vi "net_cycle_thread.vi"() -> ()   [LabVIEW 2020]
doc: "该模板用于创建生产者／消费者模式的应用程序，以事件驱动的方式，生成队列中的项。如需通过响应事件实现代码的异步执行，同时不影响用户界面的响应速度，可考虑用该模式替代“用户界面事件处理器”模式。"
uses:
  <vilib>/Instr/_visa.llb/VISA Configure Serial Port (Instr).vi
panel:
  out "转发标志1":bool
  out "发送字节数1":u32
  out "转发标志3":bool
  out "发送字节数3":u32
  out "转发标志2":bool
  out "发送字节数2":u32
  out "开启计时器 3":u32
  out "开启计时器 2":u32
  out "开启计时器":u32
  in  "关时长(ms) 3":u32
  out "数据接收 3":string
  in  "读取的字节 3":i32=500
  in  "远程端口或服务名称 3":u16=29000
  in  "远程主机地址3":string="192.168.76.100"
  in  "关时长(ms) 2":u32
  out "数据接收 2":string
  in  "读取的字节 2":i32=500
  in  "远程端口或服务名称 2":u16=28000
  in  "远程主机地址 2":string="192.168.76.200"
  in  "关时长(ms)":u32
  out "数据接收":string
  in  "读取标准码词":bool
  out "读取标准码词":string
  in  "发送数据(十六进制)":string="\u0001T\u0004"
  in  "读取的字节":i32=500
  in  "远程端口或服务名称":u16=30000
  in  "远程主机地址":string="192.168.76.172"
  in  "压缩机":bool
  in  "臭氧":bool
  in  "开时长(ms)":u32
  in  "开时长(ms) 2":u32
  in  "开时长(ms)  3":u32
  in  "开始测试":bool
  in  "风机":bool
  in  "继电器调试":bool
  in  "打开开关":bool
  in  "串口资源":refnum<visa-resource-name>
  in  "stop":bool caption="停止"
  out "错误输出":errorcluster
  out "error out":errorcluster caption="继电器板错误输入输出"
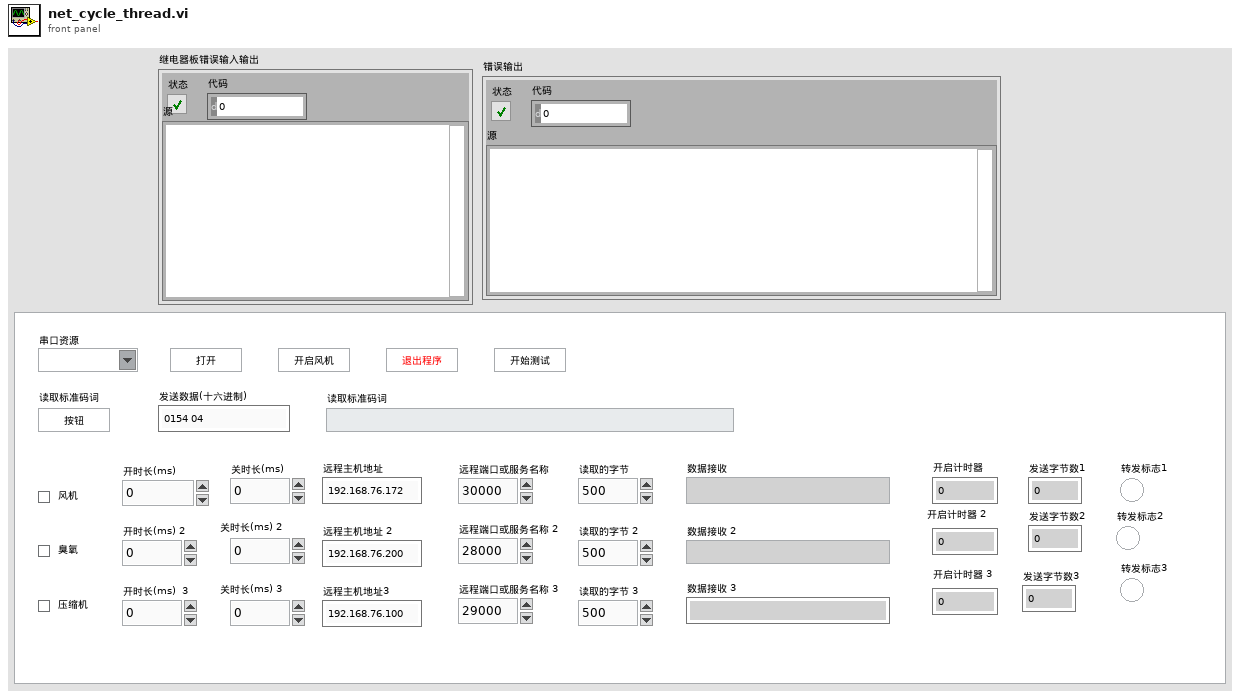
[diagram p1: front panel]
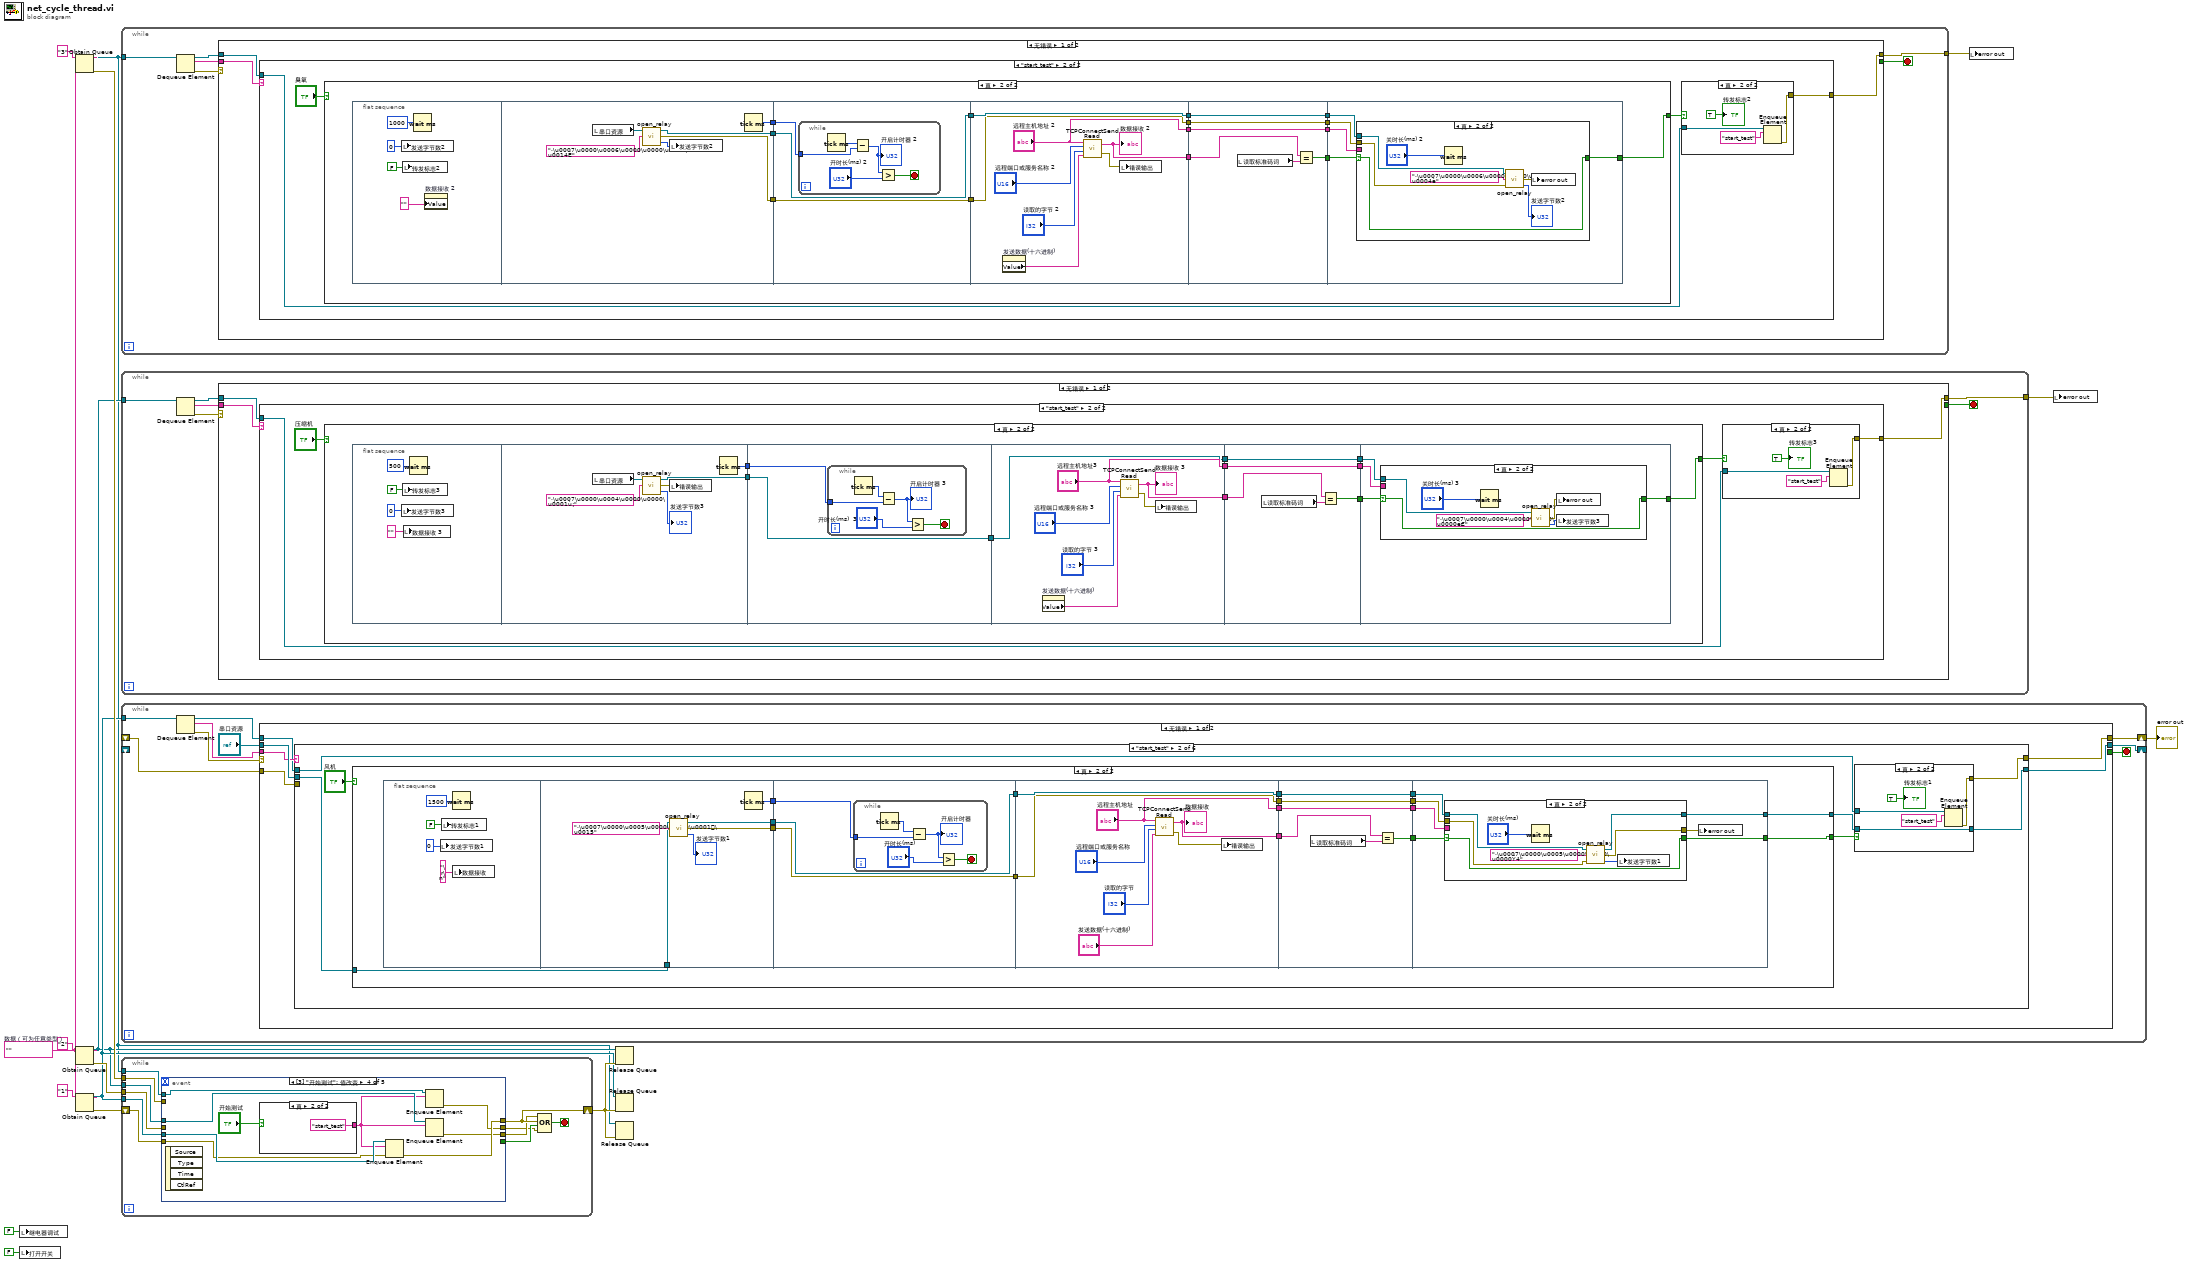
[diagram p0: block diagram]
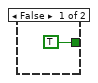
[diagram p4: hidden frame]
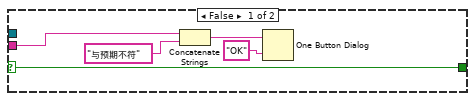
[diagram p5: hidden frame]
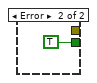
[diagram p6: hidden frame]
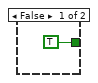
[diagram p9: hidden frame]
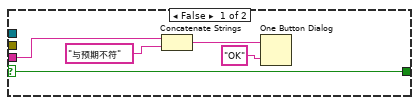
[diagram p10: hidden frame]
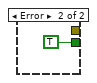
[diagram p11: hidden frame]
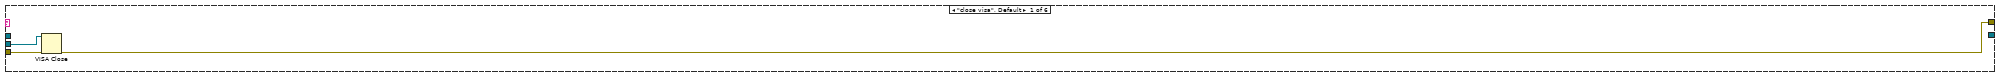
[diagram p12: hidden frame]
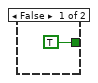
[diagram p14: hidden frame]
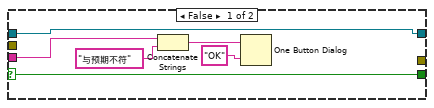
[diagram p15: hidden frame]
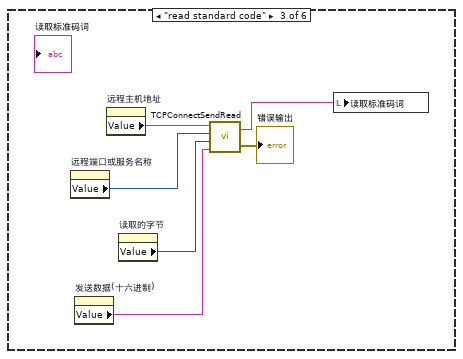
[diagram p16: hidden frame]
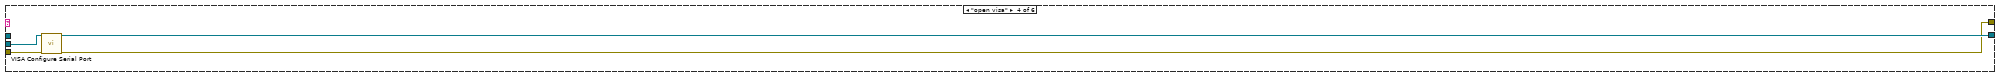
[diagram p17: hidden frame]
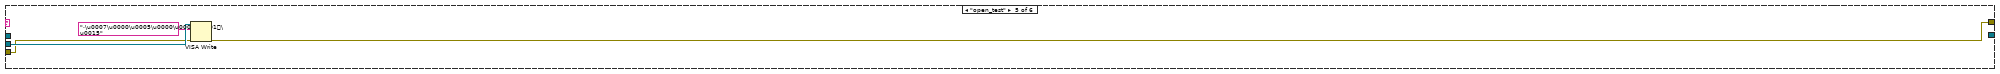
[diagram p18: hidden frame]
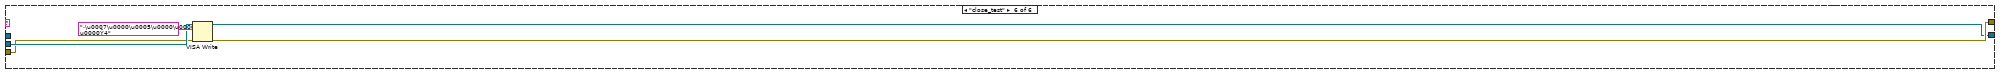
[diagram p19: hidden frame]
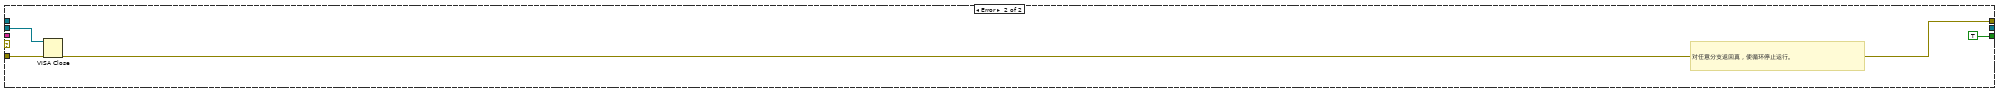
[diagram p20: hidden frame]
diagram:
  w12 = ""  # 数据（可为任意类型）
  n1 = local write "继电器调试"(FALSE ("继电器调试")) -> ()
  n2 = local write "打开开关"(FALSE ("打开开关")) -> ()
  n3 = Obtain Queue(name (unnamed)="3" ("名称（未命名）"), element data type=w12) -> (queue out=w3:refnum<queue>, error out=w11:errorcluster)  [unwired: 3 in, 1 out]
  n4 = Obtain Queue(name (unnamed)="2" ("名称（未命名）"), element data type=w12) -> (queue out=w4:refnum<queue>, error out=w10:errorcluster)  [unwired: 3 in, 1 out]
  n5 = Obtain Queue(name (unnamed)="1" ("名称（未命名）"), element data type=w12) -> (queue out=w8:refnum<queue>, error out=w16:errorcluster)  [unwired: 3 in, 1 out]
  n6 = while {
    tunnel: w3 -> [w19]
    tunnel: [w18] -> w1
    stop <- w20 stop-if-true
    n7 = Dequeue Element(queue=w19) -> (queue out=w17:refnum<queue>, element=w21:string, error out=w22:errorcluster)  [unwired: 2 in, 1 out]
    n8 = case shown="无错误" w22 {
      tunnel: w21 -> [w25 _]
      tunnel: [_ TRUE] -> w20
      tunnel: [w24 _] -> w18
      tunnel: w17 -> [w23 _]
      frame No Error {
        n9 = case shown="\"start_test\"" w25 {
          tunnel: [_ w27] -> w24
          tunnel: w23 -> [_ w26]
          frame "假", Default {
          }
          frame "start_test" {
            n10 = case shown="真" "臭氧" {
              tunnel: [TRUE w36] -> w28
              frame False {
              }
              frame True {
                n11 = flat-sequence {
                  tunnel: [w57] -> w48
                  tunnel: [w56] -> w40
                  tunnel: [w55] -> w35
                  tunnel: w48 -> [w61]
                  tunnel: [w61] -> w47
                  tunnel: [w60] -> w41
                  tunnel: w40 -> [w60]
                  tunnel: w35 -> [w59]
                  tunnel: w47 -> [w74]
                  tunnel: [w74] -> w46
                  tunnel: [w71] -> w45
                  tunnel: [w70] -> w42
                  tunnel: w41 -> [w70]
                  tunnel: ["远程主机地址 2"] -> w38
                  tunnel: w46 -> [w78]
                  tunnel: w45 -> [w80]
                  tunnel: [w78] -> w44
                  tunnel: [w77] -> w43
                  tunnel: w42 -> [w77]
                  tunnel: [w76] -> w39
                  tunnel: w38 -> [w76]
                  tunnel: [w75] -> w37
                  tunnel: w44 -> [w85]
                  tunnel: w43 -> [w84]
                  tunnel: w39 -> [w83]
                  tunnel: w37 -> [w82]
                  tunnel: [w81] -> w36
                  frame #0 {
                    n12 = local write "发送字节数2"(u32 0 ("发送字节数2")) -> ()
                    n13 = local write "转发标志2"(FALSE ("转发标志2")) -> ()
                    n14 = Wait (ms)(milliseconds to wait=u32 1000 ("等待时间（毫秒）")) -> ()  [unwired: 1 out]
                    n15 = property on="数据接收 2" class="Str"("Value"="" ("数据接收 2")) -> ()  [unwired: 2 in, 2 out]
                  }
                  frame #1 {
                    n16 = local read "串口资源"() -> (w54:refnum<visa-resource-name>)
                    n17 = call "open_relay.vi"("写入缓冲区"="·\u0007\u0000\u0006\u0000\u0000\u0001\u0014É", "VISA资源名称"=w54) -> ("返回数"=w53:u32, "错误输出"=w56:errorcluster, "VISA资源名称输出"=w57:refnum<visa-resource-name>)  [unwired: 1 in]
                    n18 = local write "发送字节数2"(w53) -> ()
                    n19 = Tick Count (ms)() -> (millisecond timer value=w55:u32)
                  }
                  frame #2 {
                    n20 = while {
                      tunnel: w59 -> [w64]
                      stop <- w65 stop-if-true
                      n21 = Tick Count (ms)() -> (millisecond timer value=w66:u32)
                      n22 = Subtract(x=w66, y=w64) -> (x-y=w63:u32)
                      "开启计时器 2" <- w63
                      n23 = Greater?(x=w63, y="开时长(ms) 2") -> (0:w65:bool)
                    }
                  }
                  frame #3 {
                    n24 = property on="发送数据(十六进制)" class="Str"() -> ("Value"=w69:string)  [unwired: 2 in, 2 out]
                    n25 = call "TCPConnectSendRead.vi"("数据输入"=w69, "读取的字节"="读取的字节 2", "远程端口或服务名称"="远程端口或服务名称 2", "地址"="远程主机地址 2") -> ("错误输出"=w67:errorcluster, "数据输出"=w71:string)
                    "数据接收 2" <- w71
                    n26 = local write "错误输出"(w67) -> ()
                  }
                  frame #4 {
                    n27 = local read "读取标准码词"() -> (w79:string)
                    n28 = Equal?(x=w80, y=w79) -> (x = y?=w75:bool)
                  }
                  frame #5 {
                    n29 = case shown="真" w82 {
                      selector: w82 -> [w86 w92]
                      tunnel: w85 -> [_ w96]
                      tunnel: w84 -> [_ w95]
                      tunnel: w83 -> [w87 _]
                      tunnel: [w86 w92] -> w81
                      frame False {
                        n30 = Concatenate Strings(w87, "与预期不符" ("字符串")) -> (w90:string)
                        n31 = One Button Dialog(message=w90, button name ("OK")="OK" ("按钮名称（“确定”）")) -> ()  [unwired: 1 out]
                      }
                      frame True {
                        n32 = Wait (ms)(milliseconds to wait="关时长(ms) 2") -> ()  [unwired: 1 out]
                        n33 = call "open_relay.vi"("错误输入（无错误）"=w95, "写入缓冲区"="·\u0007\u0000\u0006\u0000\u0000\u0000\u0004è", "VISA资源名称"=w96) -> ("返回数"=→"发送字节数2":u32, "错误输出"=w94:errorcluster)  [unwired: 1 out]
                        n34 = local write "error out"(w94) -> ()
                      }
                    }
                  }
                }
              }
            }
            n35 = case shown="真" w28 {
              tunnel: [_ w32] -> w27
              tunnel: w26 -> [_ w31]
              frame False {
              }
              frame True {
                n36 = Enqueue Element(queue=w31, element="start_test" ("元素")) -> (error out=w32:errorcluster)  [unwired: 2 in, 2 out]
                "转发标志2" <- TRUE ("转发标志2")
              }
            }
          }
        }
      }
      frame Error {
      }
    }
  }
  n37 = while {
    tunnel: w4 -> [w101]
    tunnel: [w100] -> w2
    stop <- w102 stop-if-true
    n38 = Dequeue Element(queue=w101) -> (queue out=w99:refnum<queue>, element=w103:string, error out=w104:errorcluster)  [unwired: 2 in, 1 out]
    n39 = case shown="无错误" w104 {
      tunnel: w103 -> [w107 _]
      tunnel: [_ TRUE] -> w102
      tunnel: [w106 _] -> w100
      tunnel: w99 -> [w105 _]
      frame No Error {
        n40 = case shown="\"start_test\"" w107 {
          tunnel: [_ w109] -> w106
          tunnel: w105 -> [_ w108]
          frame "假", Default {
          }
          frame "start_test" {
            n41 = case shown="真" "压缩机" {
              tunnel: [TRUE w122] -> w110
              frame False {
              }
              frame True {
                n42 = flat-sequence {
                  tunnel: [w135] -> w118
                  tunnel: [w134] -> w117
                  tunnel: [w138] -> w119
                  tunnel: w118 -> [w138]
                  tunnel: w117 -> [w137]
                  tunnel: [w146] -> w126
                  tunnel: ["远程主机地址3"] -> w123
                  tunnel: [w144] -> w120
                  tunnel: w119 -> [w144]
                  tunnel: w126 -> [w155]
                  tunnel: [w153] -> w125
                  tunnel: [w152] -> w124
                  tunnel: w123 -> [w152]
                  tunnel: [w151] -> w121
                  tunnel: w120 -> [w151]
                  tunnel: w125 -> [w159]
                  tunnel: w124 -> [w158]
                  tunnel: [w157] -> w122
                  tunnel: w121 -> [w156]
                  frame #0 {
                    n43 = local write "发送字节数3"(u32 0 ("返回数3")) -> ()
                    n44 = local write "转发标志3"(FALSE ("转发标志3")) -> ()
                    n45 = local write "数据接收 3"("" ("数据接收 3")) -> ()
                    n46 = Wait (ms)(milliseconds to wait=u32 500 ("等待时间（毫秒）")) -> ()  [unwired: 1 out]
                  }
                  frame #1 {
                    n47 = local read "串口资源"() -> (w133:refnum<visa-resource-name>)
                    n48 = call "open_relay.vi"("写入缓冲区"="·\u0007\u0000\u0004\u0000\u0000\u0001ù¡", "VISA资源名称"=w133) -> ("返回数"=→"发送字节数3":u32, "错误输出"=w132:errorcluster, "VISA资源名称输出"=w135:refnum<visa-resource-name>)  [unwired: 1 in]
                    n49 = local write "错误输出"(w132) -> ()
                    n50 = Tick Count (ms)() -> (millisecond timer value=w134:u32)
                  }
                  frame #2 {
                    n51 = while {
                      tunnel: w137 -> [w141]
                      stop <- w142 stop-if-true
                      n52 = Tick Count (ms)() -> (millisecond timer value=w143:u32)
                      n53 = Subtract(x=w143, y=w141) -> (x-y=w140:u32)
                      "开启计时器 3" <- w140
                      n54 = Greater?(x=w140, y="开时长(ms)  3") -> (0:w142:bool)
                    }
                  }
                  frame #3 {
                    n55 = property on="发送数据(十六进制)" class="Str"() -> ("Value"=w148:string)  [unwired: 2 in, 2 out]
                    n56 = call "TCPConnectSendRead.vi"("数据输入"=w148, "读取的字节"="读取的字节 3", "远程端口或服务名称"="远程端口或服务名称 3", "地址"="远程主机地址3") -> ("错误输出"=w147:errorcluster, "数据输出"=w146:string)
                    "数据接收 3" <- w146
                    n57 = local write "错误输出"(w147) -> ()
                  }
                  frame #4 {
                    n58 = local read "读取标准码词"() -> (w154:string)
                    n59 = Equal?(x=w155, y=w154) -> (x = y?=w153:bool)
                  }
                  frame #5 {
                    n60 = case shown="真" w159 {
                      selector: w159 -> [w160 w167]
                      tunnel: w158 -> [w161 _]
                      tunnel: [w160 w167] -> w157
                      tunnel: w156 -> [_ w166]
                      frame False {
                        n61 = Concatenate Strings(w161, "与预期不符" ("字符串")) -> (w162:string)
                        n62 = One Button Dialog(message=w162, button name ("OK")="OK" ("按钮名称（“确定”）")) -> ()  [unwired: 1 out]
                      }
                      frame True {
                        n63 = Wait (ms)(milliseconds to wait="关时长(ms) 3") -> ()  [unwired: 1 out]
                        n64 = call "open_relay.vi"("写入缓冲区"="·\u0007\u0000\u0004\u0000\u0000\u0000é€", "VISA资源名称"=w166) -> ("返回数"=w165:u32, "错误输出"=w169:errorcluster)  [unwired: 1 in, 1 out]
                        n65 = local write "error out"(w169) -> ()
                        n66 = local write "发送字节数3"(w165) -> ()
                      }
                    }
                  }
                }
              }
            }
            n67 = case shown="真" w110 {
              tunnel: [_ w114] -> w109
              tunnel: w108 -> [_ w113]
              frame False {
              }
              frame True {
                n68 = Enqueue Element(queue=w113, element="start_test" ("元素")) -> (error out=w114:errorcluster)  [unwired: 2 in, 2 out]
                "转发标志3" <- TRUE ("转发标志3")
              }
            }
          }
        }
      }
      frame Error {
      }
    }
  }
  n69 = while {
    tunnel: w8 -> [w180]
    shift-right: [w176] -> _
    shift-left: _ -> [_]
    shift-right: [w175] -> w15
    shift-left: _ -> [w174]
    stop <- w179 stop-if-true
    n70 = Dequeue Element(queue=w180) -> (queue out=w172:refnum<queue>, element=w177:string, error out=w178:errorcluster)  [unwired: 2 in, 1 out]
    n71 = case shown="无错误" w178 {
      tunnel: [_ TRUE] -> w179
      tunnel: w177 -> [w182 _]
      tunnel: [w186 _] -> w176
      tunnel: "串口资源" -> [w185 w293]
      tunnel: [w183 w291] -> w175
      tunnel: w174 -> [w184 w292]
      tunnel: w172 -> [w181 _]
      frame No Error {
        n72 = case shown="\"start_test\"" w182 {
          tunnel: [_ w192 _ w281 _ w287] -> w186
          tunnel: w185 -> [w189 w195 _ w278 w285 w288]
          tunnel: w184 -> [w188 _ _ w279 w282 w286]
          tunnel: [w187 w190 _ w280 w283 w290] -> w183
          tunnel: w181 -> [_ w194 _ _ _ _]
          frame "close visa", Default {
            n73 = VISA Close(VISA resource name=w189, error in (no error)=w188) -> (error out=w187:errorcluster)
          }
          frame "start_test" {
            n74 = case shown="真" "风机" {
              tunnel: w195 -> [_ w218]
              tunnel: [TRUE w213] -> w193
              tunnel: [_ w203] -> w191
              frame False {
              }
              frame True {
                n75 = flat-sequence {
                  tunnel: w218 -> [w227]
                  tunnel: [w226] -> w212
                  tunnel: [w225] -> w208
                  tunnel: [w224] -> w204
                  tunnel: w212 -> [w231]
                  tunnel: [w231] -> w211
                  tunnel: w208 -> [w230]
                  tunnel: [w230] -> w207
                  tunnel: w204 -> [w229]
                  tunnel: [w241] -> w217
                  tunnel: w211 -> [w240]
                  tunnel: [w240] -> w216
                  tunnel: ["远程主机地址"] -> w209
                  tunnel: w207 -> [w238]
                  tunnel: [w238] -> w206
                  tunnel: w217 -> [w250]
                  tunnel: w216 -> [w248]
                  tunnel: [w248] -> w215
                  tunnel: [w247] -> w214
                  tunnel: [w246] -> w210
                  tunnel: w209 -> [w246]
                  tunnel: w206 -> [w245]
                  tunnel: [w245] -> w205
                  tunnel: w215 -> [w257]
                  tunnel: w214 -> [w256]
                  tunnel: [w255] -> w213
                  tunnel: w210 -> [w254]
                  tunnel: w205 -> [w253]
                  tunnel: [w251] -> w203
                  frame #0 {
                    n76 = local write "发送字节数1"(u32 0 ("发送字节数1")) -> ()
                    n77 = local write "转发标志1"(FALSE ("转发标志1")) -> ()
                    n78 = Wait (ms)(milliseconds to wait=u32 1500 ("等待时间（毫秒）")) -> ()  [unwired: 1 out]
                    n79 = local write "数据接收"("\r\n" ("数据接收")) -> ()
                  }
                  frame #1 {
                    n80 = call "open_relay.vi"("写入缓冲区"="·\u0007\u0000\u0005\u0000\u0000\u0001\u0015", "VISA资源名称"=w227) -> ("返回数"=→"发送字节数1":u32, "错误输出"=w225:errorcluster, "VISA资源名称输出"=w226:refnum<visa-resource-name>)  [unwired: 1 in]
                    n81 = Tick Count (ms)() -> (millisecond timer value=w224:u32)
                  }
                  frame #2 {
                    n82 = while {
                      tunnel: w229 -> [w235]
                      stop <- w234 stop-if-true
                      n83 = Tick Count (ms)() -> (millisecond timer value=w236:u32)
                      n84 = Subtract(x=w236, y=w235) -> (x-y=w233:u32)
                      "开启计时器" <- w233
                      n85 = Greater?(x=w233, y="开时长(ms)") -> (0:w234:bool)
                    }
                  }
                  frame #3 {
                    n86 = call "TCPConnectSendRead.vi"("数据输入"="发送数据(十六进制)", "读取的字节"="读取的字节", "远程端口或服务名称"="远程端口或服务名称", "地址"="远程主机地址") -> ("错误输出"=w237:errorcluster, "数据输出"=w241:string)
                    "数据接收" <- w241
                    n87 = local write "错误输出"(w237) -> ()
                  }
                  frame #4 {
                    n88 = local read "读取标准码词"() -> (w249:string)
                    n89 = Equal?(x=w250, y=w249) -> (x = y?=w247:bool)
                  }
                  frame #5 {
                    n90 = case shown="真" w256 {
                      selector: w256 -> [w263 w268]
                      tunnel: w257 -> [w258 w270]
                      tunnel: [w263 w268] -> w255
                      tunnel: w254 -> [w261 _]
                      tunnel: w253 -> [_ w267]
                      tunnel: [_ w266] -> w252
                      tunnel: [w258 w265] -> w251
                      frame False {
                        n91 = Concatenate Strings(w261, "与预期不符" ("字符串")) -> (w259:string)
                        n92 = One Button Dialog(message=w259, button name ("OK")="OK" ("按钮名称（“确定”）")) -> ()  [unwired: 1 out]
                      }
                      frame True {
                        n93 = Wait (ms)(milliseconds to wait="关时长(ms)") -> ()  [unwired: 1 out]
                        n94 = call "open_relay.vi"("错误输入（无错误）"=w267, "写入缓冲区"="·\u0007\u0000\u0005\u0000\u0000\u0000Ÿ4", "VISA资源名称"=w270) -> ("返回数"=w264:u32, "错误输出"=w266:errorcluster, "VISA资源名称输出"=w265:refnum<visa-resource-name>)
                        n95 = local write "发送字节数1"(w264) -> ()
                      }
                    }
                    n96 = local write "error out"(w252) -> ()
                  }
                }
              }
            }
            n97 = case shown="真" w193 {
              tunnel: w194 -> [_ w200]
              tunnel: [_ w199] -> w192
              tunnel: w191 -> [_ w199]
              tunnel: [_ w198] -> w190
              frame False {
              }
              frame True {
                n98 = Enqueue Element(queue=w200, element="start_test" ("元素")) -> (error out=w198:errorcluster)  [unwired: 2 in, 2 out]
                "转发标志1" <- TRUE ("转发标志1")
              }
            }
          }
          frame "read standard code" {
            n99 = property on="远程端口或服务名称" class="DigNum (严格)"() -> ("Value"=w276:u16)  [unwired: 2 in, 2 out]
            n100 = property on="发送数据(十六进制)" class="Str"() -> ("Value"=w274:string)  [unwired: 2 in, 2 out]
            n101 = property on="远程主机地址" class="Str"() -> ("Value"=w275:string)  [unwired: 2 in, 2 out]
            n102 = property on="读取的字节" class="DigNum (严格)"() -> ("Value"=w277:i32)  [unwired: 2 in, 2 out]
            n103 = call "TCPConnectSendRead.vi"("数据输入"=w274, "读取的字节"=w277, "远程端口或服务名称"=w276, "地址"=w275) -> ("错误输出"=→"错误输出":errorcluster, "数据输出"=w273:string)
            n104 = local write "读取标准码词"(w273) -> ()
          }
          frame "open visa" {
            n105 = call-poly "VISA Configure Serial Port"("VISA resource name"=w278, "error in (no error)"=w279) -> ("VISA resource name out"=w281:refnum<visa-resource-name>, "error out"=w280:errorcluster)  [unwired: 12 in]
          }
          frame "open_test" {
            n106 = VISA Write(VISA resource name=w285, write buffer="·\u0007\u0000\u0005\u0000\u0000\u0001\u0015" ("写入缓冲区"), error in (no error)=w282) -> (error out=w283:errorcluster)  [unwired: 2 out]
          }
          frame "close_test" {
            n107 = VISA Write(VISA resource name=w288, write buffer="·\u0007\u0000\u0005\u0000\u0000\u0000Ÿ4" ("写入缓冲区"), error in (no error)=w286) -> (VISA resource name out=w287:refnum<visa-resource-name>, error out=w290:errorcluster)  [unwired: 1 out]
          }
        }
      }
      frame Error {
        # "对任意分支返回真，使循环停止运行。"
        n108 = VISA Close(VISA resource name=w293, error in (no error)=w292) -> (error out=w291:errorcluster)
      }
    }
  }
  "error out" <- w15
  n109 = while {
    shift-right: [w302] -> w9
    shift-left: w16 -> [w304]
    tunnel: w8 -> [w305]
    tunnel: w11 -> [w299]
    tunnel: w10 -> [w297]
    tunnel: w3 -> [w296]
    tunnel: w4 -> [w295]
    stop <- w301 stop-if-true
    n110 = event shown="[3] \"开始测试\": 值改变" {
      selector: _ -> [_ _ _ _ _]
      dyn-events: _ -> [_ _ _ _ _]
      timeout: _ -> [_ _ _ _ _]
      tunnel: w305 -> [w310 w315 w321 w329 _]
      tunnel: w304 -> [w309 _ _ w326 w335]
      tunnel: [w308 w316 w320 w330 w335] -> w302
      tunnel: [_ _ _ _ "stop"] -> w303
      tunnel: [_ _ _ w323 w334] -> w300
      tunnel: w299 -> [_ _ _ _ w334]
      tunnel: [_ _ _ w324 w333] -> w298
      tunnel: w297 -> [_ _ _ _ w333]
      tunnel: w296 -> [_ _ _ w327 _]
      tunnel: w295 -> [_ _ _ w325 _]
      event "打开开关": Value Change {
        n111 = event-data() -> ()  [unwired: 1 in, 1 out]
        n112 = case shown="假" "打开开关" {
          tunnel: ["close visa" ("element") "open visa" ("element")] -> w306
          frame False {
          }
          frame True {
          }
        }
        n113 = Enqueue Element(queue=w310, element=w306, error in (no error)=w309) -> (error out=w308:errorcluster)  [unwired: 1 in, 2 out]
      }
      event "继电器调试": Value Change {
        n114 = event-data() -> ()  [unwired: 1 in, 3 out]
        n115 = case shown="假" "继电器调试" {
          tunnel: ["close_test" ("元素") "open_test" ("元素")] -> w313
          frame False {
          }
          frame True {
          }
        }
        n116 = Enqueue Element(queue=w315, element=w313) -> (error out=w316:errorcluster)  [unwired: 2 in, 2 out]
      }
      event "读取标准码词": Value Change {
        n117 = event-data() -> ()  [unwired: 1 in, 4 out]
        n118 = Enqueue Element(queue=w321, element="read standard code" ("元素")) -> (error out=w320:errorcluster)  [unwired: 2 in, 2 out]
      }
      event "开始测试": Value Change {
        n119 = event-data() -> ()  [unwired: 1 in, 4 out]
        n120 = case shown="真" "开始测试" {
          tunnel: ["stop_test" ("元素") "start_test" ("元素")] -> w322
          frame False {
          }
          frame True {
          }
        }
        n121 = Enqueue Element(queue=w329, element=w322, error in (no error)=w326) -> (error out=w330:errorcluster)  [unwired: 1 in, 2 out]
        n122 = Enqueue Element(queue=w327, element=w322) -> (error out=w324:errorcluster)  [unwired: 2 in, 2 out]
        n123 = Enqueue Element(queue=w325, element=w322) -> (error out=w323:errorcluster)  [unwired: 2 in, 2 out]
      }
      event "stop": Value Change {
        n124 = event-data() -> ()  [unwired: 1 in, 1 out]
      }
    }
    n125 = Compound Arithmetic op=OR ("复合运算")(w300, w302, w303, w298) -> (w301:bool)
  }
  n126 = Release Queue(queue=w4, error in (no error)=w9) -> ()  [unwired: 1 in, 3 out]
  n127 = Release Queue(queue=w8, error in (no error)=w9) -> ()  [unwired: 1 in, 3 out]
  n128 = Release Queue(queue=w3, error in (no error)=w9) -> ()  [unwired: 1 in, 3 out]
  n129 = local write "error out"(w1) -> ()
  n130 = local write "error out"(w2) -> ()
